vi "Counts to Triac Direction.vi"(10 "CCW ctr":u32, 11 "CW ctr":u32) -> (2 "CW":bool, 3 "CCW":bool)   [LabVIEW 2021]
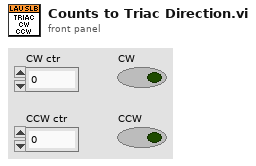
[diagram p1: front panel]
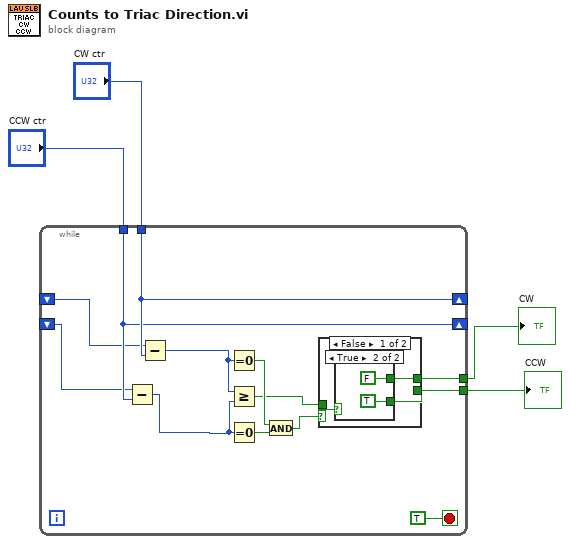
[diagram p0: block diagram]
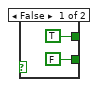
[diagram p2: hidden frame]
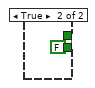
[diagram p3: hidden frame]
diagram:
  n1 = while {
    tunnel: "CCW ctr" -> [w9]
    tunnel: "CW ctr" -> [w10]
    shift-right: [w10] -> _
    shift-left: _ -> [w8]
    shift-right: [w9] -> _
    shift-left: _ -> [w7]
    tunnel: [w6] -> w2
    tunnel: [w5] -> w1
    stop <- TRUE stop-if-true
    n2 = Subtract(x=w7, y=w9) -> (x-y=w11:u32)
    n3 = Subtract(x=w8, y=w10) -> (x-y=w12:u32)
    n4 = Equal To 0?(x=w12) -> (x = 0?=w14:bool)
    n5 = Greater Or Equal?(x=w12, y=w11) -> (x >= y?=w13:bool)
    n6 = Equal To 0?(x=w11) -> (x = 0?=w15:bool)
    n7 = And(x=w14, y=w15) -> (x .and. y?=w16:bool)
    n8 = case shown="False" w16 {
      tunnel: [w20 w25] -> w6
      tunnel: [w19 w25] -> w5
      tunnel: w13 -> [w18 _]
      frame False {
        n9 = case shown="True" w18 {
          tunnel: [FALSE TRUE] -> w19
          tunnel: [TRUE FALSE] -> w20
          frame False {
          }
          frame True {
          }
        }
      }
      frame True {
        w25 = FALSE
      }
    }
  }
  "CW" <- w2
  "CCW" <- w1
